vi "Test - Draw Teapot.vi"() -> ()   [LabVIEW 2022 SP3, in "Raster.lvlib"] (continued)
{"Vertex 1"={"Position"={"x"=570.0229, "y"=136.71501, "z"=0.9889498}, "UV"={"u"=0.0, "v"=0.0}, "Colour"=12517256}, "Vertex 2"={"Position"={"x"=565.4148, "y"=132.95152, "z"=0.9889795}, "UV"={"u"=0.0, "v"=0.0}, "Colour"=12517256}, "Vertex 3"={"Position"={"x"=562.83374, "y"=124.48488, "z"=0.98841846}, "UV"={"u"=0.0, "v"=0.0}, "Colour"=12517256}, "Alpha"=0.0, "Alpha Blending Enabled"=FALSE, "Colour"=131841}, {"Vertex 1"={"Position"={"x"=413.24774, "y"=413.1011, "z"=0.988515}, "UV"={"u"=0.0, "v"=0.0}, "Colour"=12517256}, "Vertex 2"={"Position"={"x"=410.00424, "y"=412.27127, "z"=0.98889065}, "UV"={"u"=0.0, "v"=0.0}, "Colour"=12517256}, "Vertex 3"={"Position"={"x"=419.36755, "y"=411.78125, "z"=0.9889393}, "UV"={"u"=0.0, "v"=0.0}, "Colour"=12517256}, "Alpha"=0.0, "Alpha Blending Enabled"=FALSE, "Colour"=10145646}, {"Vertex 1"={"Position"={"x"=288.70093, "y"=107.824104, "z"=0.9884769}, "UV"={"u"=0.0, "v"=0.0}, "Colour"=12517256}, "Vertex 2"={"Position"={"x"=309.68015, "y"=111.224434, "z"=0.9887732}, "UV"={"u"=0.0, "v"=0.0}, "Colour"=12517256}, "Vertex 3"={"Position"={"x"=303.40628, "y"=116.389046, "z"=0.98908174}, "UV"={"u"=0.0, "v"=0.0}, "Colour"=12517256}, "Alpha"=0.0, "Alpha Blending Enabled"=FALSE, "Colour"=131841}, {"Vertex 1"={"Position"={"x"=458.76797, "y"=410.43784, "z"=0.98850775}, "UV"={"u"=0.0, "v"=0.0}, "Colour"=12517256}, "Vertex 2"={"Position"={"x"=446.6635, "y"=410.05975, "z"=0.9888252}, "UV"={"u"=0.0, "v"=0.0}, "Colour"=12517256}, "Vertex 3"={"Position"={"x"=454.95868, "y"=408.43207, "z"=0.9889912}, "UV"={"u"=0.0, "v"=0.0}, "Colour"=12517256}, "Alpha"=0.0, "Alpha Blending Enabled"=FALSE, "Colour"=9750378}, {"Vertex 1"={"Position"={"x"=234.58522, "y"=132.95152, "z"=0.9889795}, "UV"={"u"=0.0, "v"=0.0}, "Colour"=12517256}, "Vertex 2"={"Position"={"x"=229.97716, "y"=136.71501, "z"=0.9889498}, "UV"={"u"=0.0, "v"=0.0}, "Colour"=12517256}, "Vertex 3"={"Position"={"x"=232.39339, "y"=128.19644, "z"=0.98837066}, "UV"={"u"=0.0, "v"=0.0}, "Colour"=12517256}, "Alpha"=0.0, "Alpha Blending Enabled"=FALSE, "Colour"=131841}, {"Vertex 1"={"Position"={"x"=427.90894, "y"=411.00418, "z"=0.98901653}, "UV"={"u"=0.0, "v"=0.0}, "Colour"=12517256}, "Vertex 2"={"Position"={"x"=436.8227, "y"=411.41696, "z"=0.9886868}, "UV"={"u"=0.0, "v"=0.0}, "Colour"=12517256}, "Vertex 3"={"Position"={"x"=425.6105, "y"=412.44833, "z"=0.98858166}, "UV"={"u"=0.0, "v"=0.0}, "Colour"=12517256}, "Alpha"=0.0, "Alpha Blending Enabled"=FALSE, "Colour"=10079597}, {"Vertex 1"={"Position"={"x"=386.75226, "y"=413.1011, "z"=0.988515}, "UV"={"u"=0.0, "v"=0.0}, "Colour"=12517256}, "Vertex 2"={"Position"={"x"=389.99573, "y"=412.27127, "z"=0.98889065}, "UV"={"u"=0.0, "v"=0.0}, "Colour"=12517256}, "Vertex 3"={"Position"={"x"=400.0, "y"=412.4412, "z"=0.9888737}, "UV"={"u"=0.0, "v"=0.0}, "Colour"=12517256}, "Alpha"=0.0, "Alpha Blending Enabled"=FALSE, "Colour"=10211183}, {"Vertex 1"={"Position"={"x"=563.7232, "y"=388.5807, "z"=0.9889904}, "UV"={"u"=0.0, "v"=0.0}, "Colour"=12517256}, "Vertex 2"={"Position"={"x"=572.7935, "y"=370.8628, "z"=0.98893183}, "UV"={"u"=0.0, "v"=0.0}, "Colour"=12517256}, "Vertex 3"={"Position"={"x"=570.48285, "y"=374.62314, "z"=0.98834187}, "UV"={"u"=0.0, "v"=0.0}, "Colour"=12517256}, "Alpha"=0.0, "Alpha Blending Enabled"=FALSE, "Colour"=6851659}, {"Vertex 1"={"Position"={"x"=400.0, "y"=413.3279, "z"=0.9884919}, "UV"={"u"=0.0, "v"=0.0}, "Colour"=12517256}, "Vertex 2"={"Position"={"x"=400.0, "y"=412.4412, "z"=0.9888737}, "UV"={"u"=0.0, "v"=0.0}, "Colour"=12517256}, "Vertex 3"={"Position"={"x"=410.00424, "y"=412.27127, "z"=0.98889065}, "UV"={"u"=0.0, "v"=0.0}, "Colour"=12517256}, "Alpha"=0.0, "Alpha Blending Enabled"=FALSE, "Colour"=10211183}, {"Vertex 1"={"Position"={"x"=274.597, "y"=398.86298, "z"=0.98879325}, "UV"={"u"=0.0, "v"=0.0}, "Colour"=12517256}, "Vertex 2"={"Position"={"x"=286.71924, "y"=401.0599, "z"=0.98891467}, "UV"={"u"=0.0, "v"=0.0}, "Colour"=12517256}, "Vertex 3"={"Position"={"x"=293.55975, "y"=404.4099, "z"=0.98854554}, "UV"={"u"=0.0, "v"=0.0}, "Colour"=12517256}, "Alpha"=0.0, "Alpha Blending Enabled"=FALSE, "Colour"=9750378}, {"Vertex 1"={"Position"={"x"=576.8591, "y"=141.4411, "z"=0.98890555}, "UV"={"u"=0.0, "v"=0.0}, "Colour"=12517256}, "Vertex 2"={"Position"={"x"=570.0229, "y"=136.71501, "z"=0.9889498}, "UV"={"u"=0.0, "v"=0.0}, "Colour"=12517256}, "Vertex 3"={"Position"={"x"=567.6066, "y"=128.19644, "z"=0.98837066}, "UV"={"u"=0.0, "v"=0.0}, "Colour"=12517256}, "Alpha"=0.0, "Alpha Blending Enabled"=FALSE, "Colour"=131841}, {"Vertex 1"={"Position"={"x"=454.95868, "y"=408.43207, "z"=0.9889912}, "UV"={"u"=0.0, "v"=0.0}, "Colour"=12517256}, "Vertex 2"={"Position"={"x"=468.95047, "y"=408.38864, "z"=0.98872197}, "UV"={"u"=0.0, "v"=0.0}, "Colour"=12517256}, "Vertex 3"={"Position"={"x"=458.76797, "y"=410.43784, "z"=0.98850775}, "UV"={"u"=0.0, "v"=0.0}, "Colour"=12517256}, "Alpha"=0.0, "Alpha Blending Enabled"=FALSE, "Colour"=9750378}, {"Vertex 1"={"Position"={"x"=380.63242, "y"=411.78125, "z"=0.9889393}, "UV"={"u"=0.0, "v"=0.0}, "Colour"=12517256}, "Vertex 2"={"Position"={"x"=374.3895, "y"=412.44833, "z"=0.98858166}, "UV"={"u"=0.0, "v"=0.0}, "Colour"=12517256}, "Vertex 3"={"Position"={"x"=363.17734, "y"=411.41696, "z"=0.9886868}, "UV"={"u"=0.0, "v"=0.0}, "Colour"=12517256}, "Alpha"=0.0, "Alpha Blending Enabled"=FALSE, "Colour"=10079597}, {"Vertex 1"={"Position"={"x"=307.75357, "y"=405.47995, "z"=0.98874605}, "UV"={"u"=0.0, "v"=0.0}, "Colour"=12517256}, "Vertex 2"={"Position"={"x"=293.55975, "y"=404.4099, "z"=0.98854554}, "UV"={"u"=0.0, "v"=0.0}, "Colour"=12517256}, "Vertex 3"={"Position"={"x"=286.71924, "y"=401.0599, "z"=0.98891467}, "UV"={"u"=0.0, "v"=0.0}, "Colour"=12517256}, "Alpha"=0.0, "Alpha Blending Enabled"=FALSE, "Colour"=9552744}, {"Vertex 1"={"Position"={"x"=457.64166, "y"=112.87481, "z"=0.9889396}, "UV"={"u"=0.0, "v"=0.0}, "Colour"=12517256}, "Vertex 2"={"Position"={"x"=481.26578, "y"=106.39749, "z"=0.9884849}, "UV"={"u"=0.0, "v"=0.0}, "Colour"=12517256}, "Vertex 3"={"Position"={"x"=490.3199, "y"=111.224434, "z"=0.9887732}, "UV"={"u"=0.0, "v"=0.0}, "Colour"=12517256}, "Alpha"=0.0, "Alpha Blending Enabled"=FALSE, "Colour"=131841}, {"Vertex 1"={"Position"={"x"=386.10147, "y"=117.449425, "z"=0.9892527}, "UV"={"u"=0.0, "v"=0.0}, "Colour"=12517256}, "Vertex 2"={"Position"={"x"=373.09055, "y"=105.592224, "z"=0.9885072}, "UV"={"u"=0.0, "v"=0.0}, "Colour"=12517256}, "Vertex 3"={"Position"={"x"=386.07623, "y"=104.40606, "z"=0.98843676}, "UV"={"u"=0.0, "v"=0.0}, "Colour"=12517256}, "Alpha"=0.0, "Alpha Blending Enabled"=FALSE, "Colour"=131841}, {"Vertex 1"={"Position"={"x"=481.26578, "y"=106.39749, "z"=0.9884849}, "UV"={"u"=0.0, "v"=0.0}, "Colour"=12517256}, "Vertex 2"={"Position"={"x"=457.64166, "y"=112.87481, "z"=0.9889396}, "UV"={"u"=0.0, "v"=0.0}, "Colour"=12517256}, "Vertex 3"={"Position"={"x"=448.97742, "y"=109.926476, "z"=0.9887645}, "UV"={"u"=0.0, "v"=0.0}, "Colour"=12517256}, "Alpha"=0.0, "Alpha Blending Enabled"=FALSE, "Colour"=131841}, {"Vertex 1"={"Position"={"x"=245.69356, "y"=114.66924, "z"=0.9885038}, "UV"={"u"=0.0, "v"=0.0}, "Colour"=12517256}, "Vertex 2"={"Position"={"x"=253.39772, "y"=113.55681, "z"=0.98858106}, "UV"={"u"=0.0, "v"=0.0}, "Colour"=12517256}, "Vertex 3"={"Position"={"x"=250.35448, "y"=121.69325, "z"=0.9890815}, "UV"={"u"=0.0, "v"=0.0}, "Colour"=12517256}, "Alpha"=0.0, "Alpha Blending Enabled"=FALSE, "Colour"=131841}, {"Vertex 1"={"Position"={"x"=407.17038, "y"=116.87585, "z"=0.9892187}, "UV"={"u"=0.0, "v"=0.0}, "Colour"=12517256}, "Vertex 2"={"Position"={"x"=413.92374, "y"=104.40606, "z"=0.98843676}, "UV"={"u"=0.0, "v"=0.0}, "Colour"=12517256}, "Vertex 3"={"Position"={"x"=426.90945, "y"=105.592224, "z"=0.9885072}, "UV"={"u"=0.0, "v"=0.0}, "Colour"=12517256}, "Alpha"=0.0, "Alpha Blending Enabled"=FALSE, "Colour"=131841}, {"Vertex 1"={"Position"={"x"=476.9231, "y"=406.08713, "z"=0.9889625}, "UV"={"u"=0.0, "v"=0.0}, "Colour"=12517256}, "Vertex 2"={"Position"={"x"=492.24643, "y"=405.47995, "z"=0.98874605}, "UV"={"u"=0.0, "v"=0.0}, "Colour"=12517256}, "Vertex 3"={"Position"={"x"=483.04462, "y"=408.23608, "z"=0.98845065}, "UV"={"u"=0.0, "v"=0.0}, "Colour"=12517256}, "Alpha"=0.0, "Alpha Blending Enabled"=FALSE, "Colour"=9618537}, {"Vertex 1"={"Position"={"x"=551.1689, "y"=403.53403, "z"=0.9885353}, "UV"={"u"=0.0, "v"=0.0}, "Colour"=12517256}, "Vertex 2"={"Position"={"x"=549.12836, "y"=403.82065, "z"=0.98855567}, "UV"={"u"=0.0, "v"=0.0}, "Colour"=12517256}, "Vertex 3"={"Position"={"x"=552.1096, "y"=399.21527, "z"=0.9890656}, "UV"={"u"=0.0, "v"=0.0}, "Colour"=12517256}, "Alpha"=0.0, "Alpha Blending Enabled"=FALSE, "Colour"=9420646}, {"Vertex 1"={"Position"={"x"=229.97716, "y"=136.71501, "z"=0.9889498}, "UV"={"u"=0.0, "v"=0.0}, "Colour"=12517256}, "Vertex 2"={"Position"={"x"=223.14096, "y"=141.4411, "z"=0.98890555}, "UV"={"u"=0.0, "v"=0.0}, "Colour"=12517256}, "Vertex 3"={"Position"={"x"=225.2878, "y"=132.81842, "z"=0.9882995}, "UV"={"u"=0.0, "v"=0.0}, "Colour"=12517256}, "Alpha"=0.0, "Alpha Blending Enabled"=FALSE, "Colour"=131841}, {"Vertex 1"={"Position"={"x"=218.2245, "y"=353.0026, "z"=0.9888737}, "UV"={"u"=0.0, "v"=0.0}, "Colour"=12517256}, "Vertex 2"={"Position"={"x"=227.20647, "y"=370.8628, "z"=0.98893183}, "UV"={"u"=0.0, "v"=0.0}, "Colour"=12517256}, "Vertex 3"={"Position"={"x"=229.51718, "y"=374.62314, "z"=0.98834187}, "UV"={"u"=0.0, "v"=0.0}, "Colour"=12517256}, "Alpha"=0.0, "Alpha Blending Enabled"=FALSE, "Colour"=6851402}, {"Vertex 1"={"Position"={"x"=250.87166, "y"=403.82065, "z"=0.98855567}, "UV"={"u"=0.0, "v"=0.0}, "Colour"=12517256}, "Vertex 2"={"Position"={"x"=248.83113, "y"=403.53403, "z"=0.9885353}, "UV"={"u"=0.0, "v"=0.0}, "Colour"=12517256}, "Vertex 3"={"Position"={"x"=245.90259, "y"=398.88132, "z"=0.9890528}, "UV"={"u"=0.0, "v"=0.0}, "Colour"=12517256}, "Alpha"=0.0, "Alpha Blending Enabled"=FALSE, "Colour"=9420646}, {"Vertex 1"={"Position"={"x"=483.04462, "y"=408.23608, "z"=0.98845065}, "UV"={"u"=0.0, "v"=0.0}, "Colour"=12517256}, "Vertex 2"={"Position"={"x"=468.95047, "y"=408.38864, "z"=0.98872197}, "UV"={"u"=0.0, "v"=0.0}, "Colour"=12517256}, "Vertex 3"={"Position"={"x"=476.9231, "y"=406.08713, "z"=0.9889625}, "UV"={"u"=0.0, "v"=0.0}, "Colour"=12517256}, "Alpha"=0.0, "Alpha Blending Enabled"=FALSE, "Colour"=9618537}, {"Vertex 1"={"Position"={"x"=546.60223, "y"=113.55681, "z"=0.98858106}, "UV"={"u"=0.0, "v"=0.0}, "Colour"=12517256}, "Vertex 2"={"Position"={"x"=554.3064, "y"=114.66924, "z"=0.9885038}, "UV"={"u"=0.0, "v"=0.0}, "Colour"=12517256}, "Vertex 3"={"Position"={"x"=557.14923, "y"=123.16278, "z"=0.989033}, "UV"={"u"=0.0, "v"=0.0}, "Colour"=12517256}, "Alpha"=0.0, "Alpha Blending Enabled"=FALSE, "Colour"=131841}, {"Vertex 1"={"Position"={"x"=490.3199, "y"=111.224434, "z"=0.9887732}, "UV"={"u"=0.0, "v"=0.0}, "Colour"=12517256}, "Vertex 2"={"Position"={"x"=511.29907, "y"=107.824104, "z"=0.9884769}, "UV"={"u"=0.0, "v"=0.0}, "Colour"=12517256}, "Vertex 3"={"Position"={"x"=518.2786, "y"=114.2621, "z"=0.98886466}, "UV"={"u"=0.0, "v"=0.0}, "Colour"=12517256}, "Alpha"=0.0, "Alpha Blending Enabled"=FALSE, "Colour"=131841}, {"Vertex 1"={"Position"={"x"=553.5304, "y"=402.33032, "z"=0.9885116}, "UV"={"u"=0.0, "v"=0.0}, "Colour"=12517256}, "Vertex 2"={"Position"={"x"=551.1689, "y"=403.53403, "z"=0.9885353}, "UV"={"u"=0.0, "v"=0.0}, "Colour"=12517256}, "Vertex 3"={"Position"={"x"=554.0974, "y"=398.88132, "z"=0.9890528}, "UV"={"u"=0.0, "v"=0.0}, "Colour"=12517256}, "Alpha"=0.0, "Alpha Blending Enabled"=FALSE, "Colour"=9289317}, {"Vertex 1"={"Position"={"x"=513.28076, "y"=401.0599, "z"=0.98891467}, "UV"={"u"=0.0, "v"=0.0}, "Colour"=12517256}, "Vertex 2"={"Position"={"x"=525.403, "y"=398.86298, "z"=0.98879325}, "UV"={"u"=0.0, "v"=0.0}, "Colour"=12517256}, "Vertex 3"={"Position"={"x"=518.25006, "y"=402.50375, "z"=0.98837876}, "UV"={"u"=0.0, "v"=0.0}, "Colour"=12517256}, "Alpha"=0.0, "Alpha Blending Enabled"=FALSE, "Colour"=9750378}, {"Vertex 1"={"Position"={"x"=248.83113, "y"=403.53403, "z"=0.9885353}, "UV"={"u"=0.0, "v"=0.0}, "Colour"=12517256}, "Vertex 2"={"Position"={"x"=246.46959, "y"=402.33032, "z"=0.9885116}, "UV"={"u"=0.0, "v"=0.0}, "Colour"=12517256}, "Vertex 3"={"Position"={"x"=243.60504, "y"=397.66318, "z"=0.9890379}, "UV"={"u"=0.0, "v"=0.0}, "Colour"=12517256}, "Alpha"=0.0, "Alpha Blending Enabled"=FALSE, "Colour"=9289317}, {"Vertex 1"={"Position"={"x"=392.82962, "y"=116.87585, "z"=0.9892187}, "UV"={"u"=0.0, "v"=0.0}, "Colour"=12517256}, "Vertex 2"={"Position"={"x"=386.07623, "y"=104.40606, "z"=0.98843676}, "UV"={"u"=0.0, "v"=0.0}, "Colour"=12517256}, "Vertex 3"={"Position"={"x"=400.0, "y"=103.99378, "z"=0.98841226}, "UV"={"u"=0.0, "v"=0.0}, "Colour"=12517256}, "Alpha"=0.0, "Alpha Blending Enabled"=FALSE, "Colour"=131841}, {"Vertex 1"={"Position"={"x"=585.23376, "y"=147.27748, "z"=0.9888514}, "UV"={"u"=0.0, "v"=0.0}, "Colour"=12517256}, "Vertex 2"={"Position"={"x"=576.8591, "y"=141.4411, "z"=0.98890555}, "UV"={"u"=0.0, "v"=0.0}, "Colour"=12517256}, "Vertex 3"={"Position"={"x"=574.71216, "y"=132.81842, "z"=0.9882995}, "UV"={"u"=0.0, "v"=0.0}, "Colour"=12517256}, "Alpha"=0.0, "Alpha Blending Enabled"=FALSE, "Colour"=131841}, {"Vertex 1"={"Position"={"x"=400.0, "y"=116.67725, "z"=0.989207}, "UV"={"u"=0.0, "v"=0.0}, "Colour"=12517256}, "Vertex 2"={"Position"={"x"=400.0, "y"=103.99378, "z"=0.98841226}, "UV"={"u"=0.0, "v"=0.0}, "Colour"=12517256}, "Vertex 3"={"Position"={"x"=413.92374, "y"=104.40606, "z"=0.98843676}, "UV"={"u"=0.0, "v"=0.0}, "Colour"=12517256}, "Alpha"=0.0, "Alpha Blending Enabled"=FALSE, "Colour"=131841}, {"Vertex 1"={"Position"={"x"=353.3365, "y"=410.05975, "z"=0.9888252}, "UV"={"u"=0.0, "v"=0.0}, "Colour"=12517256}, "Vertex 2"={"Position"={"x"=341.23203, "y"=410.43784, "z"=0.98850775}, "UV"={"u"=0.0, "v"=0.0}, "Colour"=12517256}, "Vertex 3"={"Position"={"x"=331.04953, "y"=408.38864, "z"=0.98872197}, "UV"={"u"=0.0, "v"=0.0}, "Colour"=12517256}, "Alpha"=0.0, "Alpha Blending Enabled"=FALSE, "Colour"=9750378}, {"Vertex 1"={"Position"={"x"=572.7935, "y"=370.8628, "z"=0.98893183}, "UV"={"u"=0.0, "v"=0.0}, "Colour"=12517256}, "Vertex 2"={"Position"={"x"=581.77545, "y"=353.0026, "z"=0.9888737}, "UV"={"u"=0.0, "v"=0.0}, "Colour"=12517256}, "Vertex 3"={"Position"={"x"=579.84076, "y"=355.96957, "z"=0.98824817}, "UV"={"u"=0.0, "v"=0.0}, "Colour"=12517256}, "Alpha"=0.0, "Alpha Blending Enabled"=FALSE, "Colour"=6851402}, {"Vertex 1"={"Position"={"x"=534.80365, "y"=113.363174, "z"=0.98869914}, "UV"={"u"=0.0, "v"=0.0}, "Colour"=12517256}, "Vertex 2"={"Position"={"x"=518.2786, "y"=114.2621, "z"=0.98886466}, "UV"={"u"=0.0, "v"=0.0}, "Colour"=12517256}, "Vertex 3"={"Position"={"x"=511.29907, "y"=107.824104, "z"=0.9884769}, "UV"={"u"=0.0, "v"=0.0}, "Colour"=12517256}, "Alpha"=0.0, "Alpha Blending Enabled"=FALSE, "Colour"=131841}, {"Vertex 1"={"Position"={"x"=419.36755, "y"=411.78125, "z"=0.9889393}, "UV"={"u"=0.0, "v"=0.0}, "Colour"=12517256}, "Vertex 2"={"Position"={"x"=425.6105, "y"=412.44833, "z"=0.98858166}, "UV"={"u"=0.0, "v"=0.0}, "Colour"=12517256}, "Vertex 3"={"Position"={"x"=413.24774, "y"=413.1011, "z"=0.988515}, "UV"={"u"=0.0, "v"=0.0}, "Colour"=12517256}, "Alpha"=0.0, "Alpha Blending Enabled"=FALSE, "Colour"=10145646}, {"Vertex 1"={"Position"={"x"=556.06854, "y"=400.19006, "z"=0.9884862}, "UV"={"u"=0.0, "v"=0.0}, "Colour"=12517256}, "Vertex 2"={"Position"={"x"=553.5304, "y"=402.33032, "z"=0.9885116}, "UV"={"u"=0.0, "v"=0.0}, "Colour"=12517256}, "Vertex 3"={"Position"={"x"=556.39496, "y"=397.66318, "z"=0.9890379}, "UV"={"u"=0.0, "v"=0.0}, "Colour"=12517256}, "Alpha"=0.0, "Alpha Blending Enabled"=FALSE, "Colour"=8761951}, {"Vertex 1"={"Position"={"x"=341.23203, "y"=410.43784, "z"=0.98850775}, "UV"={"u"=0.0, "v"=0.0}, "Colour"=12517256}, "Vertex 2"={"Position"={"x"=353.3365, "y"=410.05975, "z"=0.9888252}, "UV"={"u"=0.0, "v"=0.0}, "Colour"=12517256}, "Vertex 3"={"Position"={"x"=363.17734, "y"=411.41696, "z"=0.9886868}, "UV"={"u"=0.0, "v"=0.0}, "Colour"=12517256}, "Alpha"=0.0, "Alpha Blending Enabled"=FALSE, "Colour"=9881963}, {"Vertex 1"={"Position"={"x"=246.46959, "y"=402.33032, "z"=0.9885116}, "UV"={"u"=0.0, "v"=0.0}, "Colour"=12517256}, "Vertex 2"={"Position"={"x"=243.93146, "y"=400.19006, "z"=0.9884862}, "UV"={"u"=0.0, "v"=0.0}, "Colour"=12517256}, "Vertex 3"={"Position"={"x"=241.13922, "y"=395.54843, "z"=0.9890219}, "UV"={"u"=0.0, "v"=0.0}, "Colour"=12517256}, "Alpha"=0.0, "Alpha Blending Enabled"=FALSE, "Colour"=8761951}, {"Vertex 1"={"Position"={"x"=241.30443, "y"=116.502, "z"=0.9884599}, "UV"={"u"=0.0, "v"=0.0}, "Colour"=12517256}, "Vertex 2"={"Position"={"x"=245.69356, "y"=114.66924, "z"=0.9885038}, "UV"={"u"=0.0, "v"=0.0}, "Colour"=12517256}, "Vertex 3"={"Position"={"x"=242.85078, "y"=123.16278, "z"=0.989033}, "UV"={"u"=0.0, "v"=0.0}, "Colour"=12517256}, "Alpha"=0.0, "Alpha Blending Enabled"=FALSE, "Colour"=131841}, {"Vertex 1"={"Position"={"x"=389.99573, "y"=412.27127, "z"=0.98889065}, "UV"={"u"=0.0, "v"=0.0}, "Colour"=12517256}, "Vertex 2"={"Position"={"x"=386.75226, "y"=413.1011, "z"=0.988515}, "UV"={"u"=0.0, "v"=0.0}, "Colour"=12517256}, "Vertex 3"={"Position"={"x"=374.3895, "y"=412.44833, "z"=0.98858166}, "UV"={"u"=0.0, "v"=0.0}, "Colour"=12517256}, "Alpha"=0.0, "Alpha Blending Enabled"=FALSE, "Colour"=10145646}, {"Vertex 1"={"Position"={"x"=554.3064, "y"=114.66924, "z"=0.9885038}, "UV"={"u"=0.0, "v"=0.0}, "Colour"=12517256}, "Vertex 2"={"Position"={"x"=558.6956, "y"=116.502, "z"=0.9884599}, "UV"={"u"=0.0, "v"=0.0}, "Colour"=12517256}, "Vertex 3"={"Position"={"x"=561.4089, "y"=125.13941, "z"=0.98900545}, "UV"={"u"=0.0, "v"=0.0}, "Colour"=12517256}, "Alpha"=0.0, "Alpha Blending Enabled"=FALSE, "Colour"=131841}, {"Vertex 1"={"Position"={"x"=223.14096, "y"=141.4411, "z"=0.98890555}, "UV"={"u"=0.0, "v"=0.0}, "Colour"=12517256}, "Vertex 2"={"Position"={"x"=214.76619, "y"=147.27748, "z"=0.9888514}, "UV"={"u"=0.0, "v"=0.0}, "Colour"=12517256}, "Vertex 3"={"Position"={"x"=216.54234, "y"=138.55649, "z"=0.9882119}, "UV"={"u"=0.0, "v"=0.0}, "Colour"=12517256}, "Alpha"=0.0, "Alpha Blending Enabled"=FALSE, "Colour"=131841}, {"Vertex 1"={"Position"={"x"=558.6366, "y"=397.0934, "z"=0.9884605}, "UV"={"u"=0.0, "v"=0.0}, "Colour"=12517256}, "Vertex 2"={"Position"={"x"=556.06854, "y"=400.19006, "z"=0.9884862}, "UV"={"u"=0.0, "v"=0.0}, "Colour"=12517256}, "Vertex 3"={"Position"={"x"=558.8608, "y"=395.54843, "z"=0.9890219}, "UV"={"u"=0.0, "v"=0.0}, "Colour"=12517256}, "Alpha"=0.0, "Alpha Blending Enabled"=FALSE, "Colour"=8037463}, {"Vertex 1"={"Position"={"x"=243.93146, "y"=400.19006, "z"=0.9884862}, "UV"={"u"=0.0, "v"=0.0}, "Colour"=12517256}, "Vertex 2"={"Position"={"x"=241.36343, "y"=397.0934, "z"=0.9884605}, "UV"={"u"=0.0, "v"=0.0}, "Colour"=12517256}, "Vertex 3"={"Position"={"x"=238.64832, "y"=392.52478, "z"=0.9890058}, "UV"={"u"=0.0, "v"=0.0}, "Colour"=12517256}, "Alpha"=0.0, "Alpha Blending Enabled"=FALSE, "Colour"=8037463}, {"Vertex 1"={"Position"={"x"=209.52173, "y"=335.05237, "z"=0.9888175}, "UV"={"u"=0.0, "v"=0.0}, "Colour"=12517256}, "Vertex 2"={"Position"={"x"=218.2245, "y"=353.0026, "z"=0.9888737}, "UV"={"u"=0.0, "v"=0.0}, "Colour"=12517256}, "Vertex 3"={"Position"={"x"=220.15924, "y"=355.96957, "z"=0.98824817}, "UV"={"u"=0.0, "v"=0.0}, "Colour"=12517256}, "Alpha"=0.0, "Alpha Blending Enabled"=FALSE, "Colour"=6719817}, {"Vertex 1"={"Position"={"x"=330.50076, "y"=102.06894, "z"=0.9882263}, "UV"={"u"=0.0, "v"=0.0}, "Colour"=12517256}, "Vertex 2"={"Position"={"x"=351.02258, "y"=109.926476, "z"=0.9887645}, "UV"={"u"=0.0, "v"=0.0}, "Colour"=12517256}, "Vertex 3"={"Position"={"x"=342.35834, "y"=112.87481, "z"=0.9889396}, "UV"={"u"=0.0, "v"=0.0}, "Colour"=12517256}, "Alpha"=0.0, "Alpha Blending Enabled"=FALSE, "Colour"=131841}, {"Vertex 1"={"Position"={"x"=331.04953, "y"=408.38864, "z"=0.98872197}, "UV"={"u"=0.0, "v"=0.0}, "Colour"=12517256}, "Vertex 2"={"Position"={"x"=316.9554, "y"=408.23608, "z"=0.98845065}, "UV"={"u"=0.0, "v"=0.0}, "Colour"=12517256}, "Vertex 3"={"Position"={"x"=307.75357, "y"=405.47995, "z"=0.98874605}, "UV"={"u"=0.0, "v"=0.0}, "Colour"=12517256}, "Alpha"=0.0, "Alpha Blending Enabled"=FALSE, "Colour"=9618537}, {"Vertex 1"={"Position"={"x"=239.35435, "y"=118.843834, "z"=0.98844033}, "UV"={"u"=0.0, "v"=0.0}, "Colour"=12517256}, "Vertex 2"={"Position"={"x"=241.30443, "y"=116.502, "z"=0.9884599}, "UV"={"u"=0.0, "v"=0.0}, "Colour"=12517256}, "Vertex 3"={"Position"={"x"=238.5911, "y"=125.13941, "z"=0.98900545}, "UV"={"u"=0.0, "v"=0.0}, "Colour"=12517256}, "Alpha"=0.0, "Alpha Blending Enabled"=FALSE, "Colour"=131841}, {"Vertex 1"={"Position"={"x"=561.08514, "y"=393.02213, "z"=0.988436}, "UV"={"u"=0.0, "v"=0.0}, "Colour"=12517256}, "Vertex 2"={"Position"={"x"=558.6366, "y"=397.0934, "z"=0.9884605}, "UV"={"u"=0.0, "v"=0.0}, "Colour"=12517256}, "Vertex 3"={"Position"={"x"=561.3517, "y"=392.52478, "z"=0.9890058}, "UV"={"u"=0.0, "v"=0.0}, "Colour"=12517256}, "Alpha"=0.0, "Alpha Blending Enabled"=FALSE, "Colour"=7246927}, {"Vertex 1"={"Position"={"x"=410.00424, "y"=412.27127, "z"=0.98889065}, "UV"={"u"=0.0, "v"=0.0}, "Colour"=12517256}, "Vertex 2"={"Position"={"x"=413.24774, "y"=413.1011, "z"=0.988515}, "UV"={"u"=0.0, "v"=0.0}, "Colour"=12517256}, "Vertex 3"={"Position"={"x"=400.0, "y"=413.3279, "z"=0.9884919}, "UV"={"u"=0.0, "v"=0.0}, "Colour"=12517256}, "Alpha"=0.0, "Alpha Blending Enabled"=FALSE, "Colour"=10211183}, {"Vertex 1"={"Position"={"x"=558.6956, "y"=116.502, "z"=0.9884599}, "UV"={"u"=0.0, "v"=0.0}, "Colour"=12517256}, "Vertex 2"={"Position"={"x"=560.6457, "y"=118.843834, "z"=0.98844033}, "UV"={"u"=0.0, "v"=0.0}, "Colour"=12517256}, "Vertex 3"={"Position"={"x"=563.29785, "y"=127.47084, "z"=0.9889933}, "UV"={"u"=0.0, "v"=0.0}, "Colour"=12517256}, "Alpha"=0.0, "Alpha Blending Enabled"=FALSE, "Colour"=131841}, {"Vertex 1"={"Position"={"x"=241.36343, "y"=397.0934, "z"=0.9884605}, "UV"={"u"=0.0, "v"=0.0}, "Colour"=12517256}, "Vertex 2"={"Position"={"x"=238.91487, "y"=393.02213, "z"=0.988436}, "UV"={"u"=0.0, "v"=0.0}, "Colour"=12517256}, "Vertex 3"={"Position"={"x"=236.27676, "y"=388.5807, "z"=0.9889904}, "UV"={"u"=0.0, "v"=0.0}, "Colour"=12517256}, "Alpha"=0.0, "Alpha Blending Enabled"=FALSE, "Colour"=7246927}, {"Vertex 1"={"Position"={"x"=266.35956, "y"=395.62842, "z"=0.98871076}, "UV"={"u"=0.0, "v"=0.0}, "Colour"=12517256}, "Vertex 2"={"Position"={"x"=274.597, "y"=398.86298, "z"=0.98879325}, "UV"={"u"=0.0, "v"=0.0}, "Colour"=12517256}, "Vertex 3"={"Position"={"x"=281.74997, "y"=402.50375, "z"=0.98837876}, "UV"={"u"=0.0, "v"=0.0}, "Colour"=12517256}, "Alpha"=0.0, "Alpha Blending Enabled"=FALSE, "Colour"=10013549}, {"Vertex 1"={"Position"={"x"=400.0, "y"=412.4412, "z"=0.9888737}, "UV"={"u"=0.0, "v"=0.0}, "Colour"=12517256}, "Vertex 2"={"Position"={"x"=400.0, "y"=413.3279, "z"=0.9884919}, "UV"={"u"=0.0, "v"=0.0}, "Colour"=12517256}, "Vertex 3"={"Position"={"x"=386.75226, "y"=413.1011, "z"=0.988515}, "UV"={"u"=0.0, "v"=0.0}, "Colour"=12517256}, "Alpha"=0.0, "Alpha Blending Enabled"=FALSE, "Colour"=10211183}, {"Vertex 1"={"Position"={"x"=238.91487, "y"=121.48155, "z"=0.988436}, "UV"={"u"=0.0, "v"=0.0}, "Colour"=12517256}, "Vertex 2"={"Position"={"x"=239.35435, "y"=118.843834, "z"=0.98844033}, "UV"={"u"=0.0, "v"=0.0}, "Colour"=12517256}, "Vertex 3"={"Position"={"x"=236.70218, "y"=127.47084, "z"=0.9889933}, "UV"={"u"=0.0, "v"=0.0}, "Colour"=12517256}, "Alpha"=0.0, "Alpha Blending Enabled"=FALSE, "Colour"=1976342}, {"Vertex 1"={"Position"={"x"=560.6457, "y"=118.843834, "z"=0.98844033}, "UV"={"u"=0.0, "v"=0.0}, "Colour"=12517256}, "Vertex 2"={"Position"={"x"=561.08514, "y"=121.48155, "z"=0.988436}, "UV"={"u"=0.0, "v"=0.0}, "Colour"=12517256}, "Vertex 3"={"Position"={"x"=563.7232, "y"=130.00505, "z"=0.9889904}, "UV"={"u"=0.0, "v"=0.0}, "Colour"=12517256}, "Alpha"=0.0, "Alpha Blending Enabled"=FALSE, "Colour"=1976342}, {"Vertex 1"={"Position"={"x"=594.4404, "y"=154.37106, "z"=0.98879194}, "UV"={"u"=0.0, "v"=0.0}, "Colour"=12517256}, "Vertex 2"={"Position"={"x"=585.23376, "y"=147.27748, "z"=0.9888514}, "UV"={"u"=0.0, "v"=0.0}, "Colour"=12517256}, "Vertex 3"={"Position"={"x"=583.45764, "y"=138.55649, "z"=0.9882119}, "UV"={"u"=0.0, "v"=0.0}, "Colour"=12517256}, "Alpha"=0.0, "Alpha Blending Enabled"=FALSE, "Colour"=131841}, {"Vertex 1"={"Position"={"x"=581.77545, "y"=353.0026, "z"=0.9888737}, "UV"={"u"=0.0, "v"=0.0}, "Colour"=12517256}, "Vertex 2"={"Position"={"x"=590.4783, "y"=335.05237, "z"=0.9888175}, "UV"={"u"=0.0, "v"=0.0}, "Colour"=12517256}, "Vertex 3"={"Position"={"x"=588.9574, "y"=337.11398, "z"=0.98815686}, "UV"={"u"=0.0, "v"=0.0}, "Colour"=12517256}, "Alpha"=0.0, "Alpha Blending Enabled"=FALSE, "Colour"=6719817}, {"Vertex 1"={"Position"={"x"=237.16626, "y"=124.48488, "z"=0.98841846}, "UV"={"u"=0.0, "v"=0.0}, "Colour"=12517256}, "Vertex 2"={"Position"={"x"=238.91487, "y"=121.48155, "z"=0.988436}, "UV"={"u"=0.0, "v"=0.0}, "Colour"=12517256}, "Vertex 3"={"Position"={"x"=236.27676, "y"=130.00505, "z"=0.9889904}, "UV"={"u"=0.0, "v"=0.0}, "Colour"=12517256}, "Alpha"=0.0, "Alpha Blending Enabled"=FALSE, "Colour"=131841}, {"Vertex 1"={"Position"={"x"=446.5233, "y"=412.15842, "z"=0.988328}, "UV"={"u"=0.0, "v"=0.0}, "Colour"=12517256}, "Vertex 2"={"Position"={"x"=436.8227, "y"=411.41696, "z"=0.9886868}, "UV"={"u"=0.0, "v"=0.0}, "Colour"=12517256}, "Vertex 3"={"Position"={"x"=446.6635, "y"=410.05975, "z"=0.9888252}, "UV"={"u"=0.0, "v"=0.0}, "Colour"=12517256}, "Alpha"=0.0, "Alpha Blending Enabled"=FALSE, "Colour"=9881963}, {"Vertex 1"={"Position"={"x"=518.25006, "y"=402.50375, "z"=0.98837876}, "UV"={"u"=0.0, "v"=0.0}, "Colour"=12517256}, "Vertex 2"={"Position"={"x"=506.44025, "y"=404.4099, "z"=0.98854554}, "UV"={"u"=0.0, "v"=0.0}, "Colour"=12517256}, "Vertex 3"={"Position"={"x"=513.28076, "y"=401.0599, "z"=0.98891467}, "UV"={"u"=0.0, "v"=0.0}, "Colour"=12517256}, "Alpha"=0.0, "Alpha Blending Enabled"=FALSE, "Colour"=9750378}, {"Vertex 1"={"Position"={"x"=561.08514, "y"=121.48155, "z"=0.988436}, "UV"={"u"=0.0, "v"=0.0}, "Colour"=12517256}, "Vertex 2"={"Position"={"x"=562.83374, "y"=124.48488, "z"=0.98841846}, "UV"={"u"=0.0, "v"=0.0}, "Colour"=12517256}, "Vertex 3"={"Position"={"x"=565.4148, "y"=132.95152, "z"=0.9889795}, "UV"={"u"=0.0, "v"=0.0}, "Colour"=12517256}, "Alpha"=0.0, "Alpha Blending Enabled"=FALSE, "Colour"=131841}, {"Vertex 1"={"Position"={"x"=281.7214, "y"=114.2621, "z"=0.98886466}, "UV"={"u"=0.0, "v"=0.0}, "Colour"=12517256}, "Vertex 2"={"Position"={"x"=265.19638, "y"=113.363174, "z"=0.98869914}, "UV"={"u"=0.0, "v"=0.0}, "Colour"=12517256}, "Vertex 3"={"Position"={"x"=272.53372, "y"=105.9543, "z"=0.9882486}, "UV"={"u"=0.0, "v"=0.0}, "Colour"=12517256}, "Alpha"=0.0, "Alpha Blending Enabled"=FALSE, "Colour"=131841}, {"Vertex 1"={"Position"={"x"=525.403, "y"=398.86298, "z"=0.98879325}, "UV"={"u"=0.0, "v"=0.0}, "Colour"=12517256}, "Vertex 2"={"Position"={"x"=533.64044, "y"=395.62842, "z"=0.98871076}, "UV"={"u"=0.0, "v"=0.0}, "Colour"=12517256}, "Vertex 3"={"Position"={"x"=526.323, "y"=399.39044, "z"=0.9882647}, "UV"={"u"=0.0, "v"=0.0}, "Colour"=12517256}, "Alpha"=0.0, "Alpha Blending Enabled"=FALSE, "Colour"=10013549}, {"Vertex 1"={"Position"={"x"=232.39339, "y"=128.19644, "z"=0.98837066}, "UV"={"u"=0.0, "v"=0.0}, "Colour"=12517256}, "Vertex 2"={"Position"={"x"=237.16626, "y"=124.48488, "z"=0.98841846}, "UV"={"u"=0.0, "v"=0.0}, "Colour"=12517256}, "Vertex 3"={"Position"={"x"=234.58522, "y"=132.95152, "z"=0.9889795}, "UV"={"u"=0.0, "v"=0.0}, "Colour"=12517256}, "Alpha"=0.0, "Alpha Blending Enabled"=FALSE, "Colour"=131841}, {"Vertex 1"={"Position"={"x"=570.48285, "y"=374.62314, "z"=0.98834187}, "UV"={"u"=0.0, "v"=0.0}, "Colour"=12517256}, "Vertex 2"={"Position"={"x"=561.08514, "y"=393.02213, "z"=0.988436}, "UV"={"u"=0.0, "v"=0.0}, "Colour"=12517256}, "Vertex 3"={"Position"={"x"=563.7232, "y"=388.5807, "z"=0.9889904}, "UV"={"u"=0.0, "v"=0.0}, "Colour"=12517256}, "Alpha"=0.0, "Alpha Blending Enabled"=FALSE, "Colour"=6851659}, {"Vertex 1"={"Position"={"x"=214.76619, "y"=147.27748, "z"=0.9888514}, "UV"={"u"=0.0, "v"=0.0}, "Colour"=12517256}, "Vertex 2"={"Position"={"x"=205.55954, "y"=154.37106, "z"=0.98879194}, "UV"={"u"=0.0, "v"=0.0}, "Colour"=12517256}, "Vertex 3"={"Position"={"x"=206.8759, "y"=145.61699, "z"=0.9881152}, "UV"={"u"=0.0, "v"=0.0}, "Colour"=12517256}, "Alpha"=0.0, "Alpha Blending Enabled"=FALSE, "Colour"=131841}, {"Vertex 1"={"Position"={"x"=293.55975, "y"=404.4099, "z"=0.98854554}, "UV"={"u"=0.0, "v"=0.0}, "Colour"=12517256}, "Vertex 2"={"Position"={"x"=307.75357, "y"=405.47995, "z"=0.98874605}, "UV"={"u"=0.0, "v"=0.0}, "Colour"=12517256}, "Vertex 3"={"Position"={"x"=316.9554, "y"=408.23608, "z"=0.98845065}, "UV"={"u"=0.0, "v"=0.0}, "Colour"=12517256}, "Alpha"=0.0, "Alpha Blending Enabled"=FALSE, "Colour"=9750378}, {"Vertex 1"={"Position"={"x"=562.83374, "y"=124.48488, "z"=0.98841846}, "UV"={"u"=0.0, "v"=0.0}, "Colour"=12517256}, "Vertex 2"={"Position"={"x"=567.6066, "y"=128.19644, "z"=0.98837066}, "UV"={"u"=0.0, "v"=0.0}, "Colour"=12517256}, "Vertex 3"={"Position"={"x"=570.0229, "y"=136.71501, "z"=0.9889498}, "UV"={"u"=0.0, "v"=0.0}, "Colour"=12517256}, "Alpha"=0.0, "Alpha Blending Enabled"=FALSE, "Colour"=131841}, {"Vertex 1"={"Position"={"x"=201.29657, "y"=317.0733, "z"=0.9887643}, "UV"={"u"=0.0, "v"=0.0}, "Colour"=12517256}, "Vertex 2"={"Position"={"x"=209.52173, "y"=335.05237, "z"=0.9888175}, "UV"={"u"=0.0, "v"=0.0}, "Colour"=12517256}, "Vertex 3"={"Position"={"x"=211.0426, "y"=337.11398, "z"=0.98815686}, "UV"={"u"=0.0, "v"=0.0}, "Colour"=12517256}, "Alpha"=0.0, "Alpha Blending Enabled"=FALSE, "Colour"=6587976}, {"Vertex 1"={"Position"={"x"=511.29907, "y"=107.824104, "z"=0.9884769}, "UV"={"u"=0.0, "v"=0.0}, "Colour"=12517256}, "Vertex 2"={"Position"={"x"=490.3199, "y"=111.224434, "z"=0.9887732}, "UV"={"u"=0.0, "v"=0.0}, "Colour"=12517256}, "Vertex 3"={"Position"={"x"=481.26578, "y"=106.39749, "z"=0.9884849}, "UV"={"u"=0.0, "v"=0.0}, "Colour"=12517256}, "Alpha"=0.0, "Alpha Blending Enabled"=FALSE, "Colour"=131841}, {"Vertex 1"={"Position"={"x"=293.55975, "y"=404.4099, "z"=0.98854554}, "UV"={"u"=0.0, "v"=0.0}, "Colour"=12517256}, "Vertex 2"={"Position"={"x"=281.74997, "y"=402.50375, "z"=0.98837876}, "UV"={"u"=0.0, "v"=0.0}, "Colour"=12517256}, "Vertex 3"={"Position"={"x"=274.597, "y"=398.86298, "z"=0.98879325}, "UV"={"u"=0.0, "v"=0.0}, "Colour"=12517256}, "Alpha"=0.0, "Alpha Blending Enabled"=FALSE, "Colour"=9750378}, {"Vertex 1"={"Position"={"x"=238.91487, "y"=393.02213, "z"=0.988436}, "UV"={"u"=0.0, "v"=0.0}, "Colour"=12517256}, "Vertex 2"={"Position"={"x"=229.51718, "y"=374.62314, "z"=0.98834187}, "UV"={"u"=0.0, "v"=0.0}, "Colour"=12517256}, "Vertex 3"={"Position"={"x"=227.20647, "y"=370.8628, "z"=0.98893183}, "UV"={"u"=0.0, "v"=0.0}, "Colour"=12517256}, "Alpha"=0.0, "Alpha Blending Enabled"=FALSE, "Colour"=6851659}, {"Vertex 1"={"Position"={"x"=316.9554, "y"=408.23608, "z"=0.98845065}, "UV"={"u"=0.0, "v"=0.0}, "Colour"=12517256}, "Vertex 2"={"Position"={"x"=331.04953, "y"=408.38864, "z"=0.98872197}, "UV"={"u"=0.0, "v"=0.0}, "Colour"=12517256}, "Vertex 3"={"Position"={"x"=341.23203, "y"=410.43784, "z"=0.98850775}, "UV"={"u"=0.0, "v"=0.0}, "Colour"=12517256}, "Alpha"=0.0, "Alpha Blending Enabled"=FALSE, "Colour"=9815914}, {"Vertex 1"={"Position"={"x"=446.6635, "y"=410.05975, "z"=0.9888252}, "UV"={"u"=0.0, "v"=0.0}, "Colour"=12517256}, "Vertex 2"={"Position"={"x"=458.76797, "y"=410.43784, "z"=0.98850775}, "UV"={"u"=0.0, "v"=0.0}, "Colour"=12517256}, "Vertex 3"={"Position"={"x"=446.5233, "y"=412.15842, "z"=0.988328}, "UV"={"u"=0.0, "v"=0.0}, "Colour"=12517256}, "Alpha"=0.0, "Alpha Blending Enabled"=FALSE, "Colour"=9881963}, {"Vertex 1"={"Position"={"x"=263.33197, "y"=391.06378, "z"=0.9886805}, "UV"={"u"=0.0, "v"=0.0}, "Colour"=12517256}, "Vertex 2"={"Position"={"x"=266.35956, "y"=395.62842, "z"=0.98871076}, "UV"={"u"=0.0, "v"=0.0}, "Colour"=12517256}, "Vertex 3"={"Position"={"x"=273.677, "y"=399.39044, "z"=0.9882647}, "UV"={"u"=0.0, "v"=0.0}, "Colour"=12517256}, "Alpha"=0.0, "Alpha Blending Enabled"=FALSE, "Colour"=8630366}, {"Vertex 1"={"Position"={"x"=590.4783, "y"=335.05237, "z"=0.9888175}, "UV"={"u"=0.0, "v"=0.0}, "Colour"=12517256}, "Vertex 2"={"Position"={"x"=598.7034, "y"=317.0733, "z"=0.9887643}, "UV"={"u"=0.0, "v"=0.0}, "Colour"=12517256}, "Vertex 3"={"Position"={"x"=597.6187, "y"=318.1235, "z"=0.98807013}, "UV"={"u"=0.0, "v"=0.0}, "Colour"=12517256}, "Alpha"=0.0, "Alpha Blending Enabled"=FALSE, "Colour"=6587976}, {"Vertex 1"={"Position"={"x"=342.35834, "y"=112.87481, "z"=0.9889396}, "UV"={"u"=0.0, "v"=0.0}, "Colour"=12517256}, "Vertex 2"={"Position"={"x"=318.7342, "y"=106.39749, "z"=0.9884849}, "UV"={"u"=0.0, "v"=0.0}, "Colour"=12517256}, "Vertex 3"={"Position"={"x"=330.50076, "y"=102.06894, "z"=0.9882263}, "UV"={"u"=0.0, "v"=0.0}, "Colour"=12517256}, "Alpha"=0.0, "Alpha Blending Enabled"=FALSE, "Colour"=131841}, {"Vertex 1"={"Position"={"x"=603.7455, "y"=162.86359, "z"=0.98873174}, "UV"={"u"=0.0, "v"=0.0}, "Colour"=12517256}, "Vertex 2"={"Position"={"x"=594.4404, "y"=154.37106, "z"=0.98879194}, "UV"={"u"=0.0, "v"=0.0}, "Colour"=12517256}, "Vertex 3"={"Position"={"x"=593.1241, "y"=145.61699, "z"=0.9881152}, "UV"={"u"=0.0, "v"=0.0}, "Colour"=12517256}, "Alpha"=0.0, "Alpha Blending Enabled"=FALSE, "Colour"=131841}, {"Vertex 1"={"Position"={"x"=225.2878, "y"=132.81842, "z"=0.9882995}, "UV"={"u"=0.0, "v"=0.0}, "Colour"=12517256}, "Vertex 2"={"Position"={"x"=232.39339, "y"=128.19644, "z"=0.98837066}, "UV"={"u"=0.0, "v"=0.0}, "Colour"=12517256}, "Vertex 3"={"Position"={"x"=229.97716, "y"=136.71501, "z"=0.9889498}, "UV"={"u"=0.0, "v"=0.0}, "Colour"=12517256}, "Alpha"=0.0, "Alpha Blending Enabled"=FALSE, "Colour"=131841}, {"Vertex 1"={"Position"={"x"=533.64044, "y"=395.62842, "z"=0.98871076}, "UV"={"u"=0.0, "v"=0.0}, "Colour"=12517256}, "Vertex 2"={"Position"={"x"=536.668, "y"=391.06378, "z"=0.9886805}, "UV"={"u"=0.0, "v"=0.0}, "Colour"=12517256}, "Vertex 3"={"Position"={"x"=529.3001, 
